vi "test_TrajectoryDL091126GenericVoxel.vi"() -> ()   [LabVIEW 2010, in "TrajectoryDL091126GenericVoxel.lvclass"]
uses:
  TrajectoryDL091126GenericVoxel.lvclass
  <vilib>/Native 3D Graph/xcontrol/3DPC_SurfacePlot.xctl
  transformation_parameters.ctl
  common/classes/SpaceVector/SpaceVector/SpaceVector.lvclass
  common/enumerations/x_y_z_enumeration.ctl
  common/enumerations/functional_global_action_enum.ctl
panel:
  in  "centerButton":bool
  in  "z offset":dbl[unit](slide)
  in  "y offset":dbl[unit](slide)
  in  "x offset":dbl[unit](slide)
  in  "number of voxels":i32=20
  in  "createPixelsButton":bool
  in  "equallyDistributeButton":bool
  out "time needed [ms]":u32
  in  "tilt angle":dbl[unit](slide)
  in  "rotation angle":dbl[unit](slide)
  in  "scale factor":dbl(slide)=1.0 scale=1.0..10.0
  out "3D Graph":refnum<class "Base Datatype.lvclass">[](xcontrol)
  in  "stopButton":bool
  # "Test Suite for TrajectoryDL091126GenericVoxel"
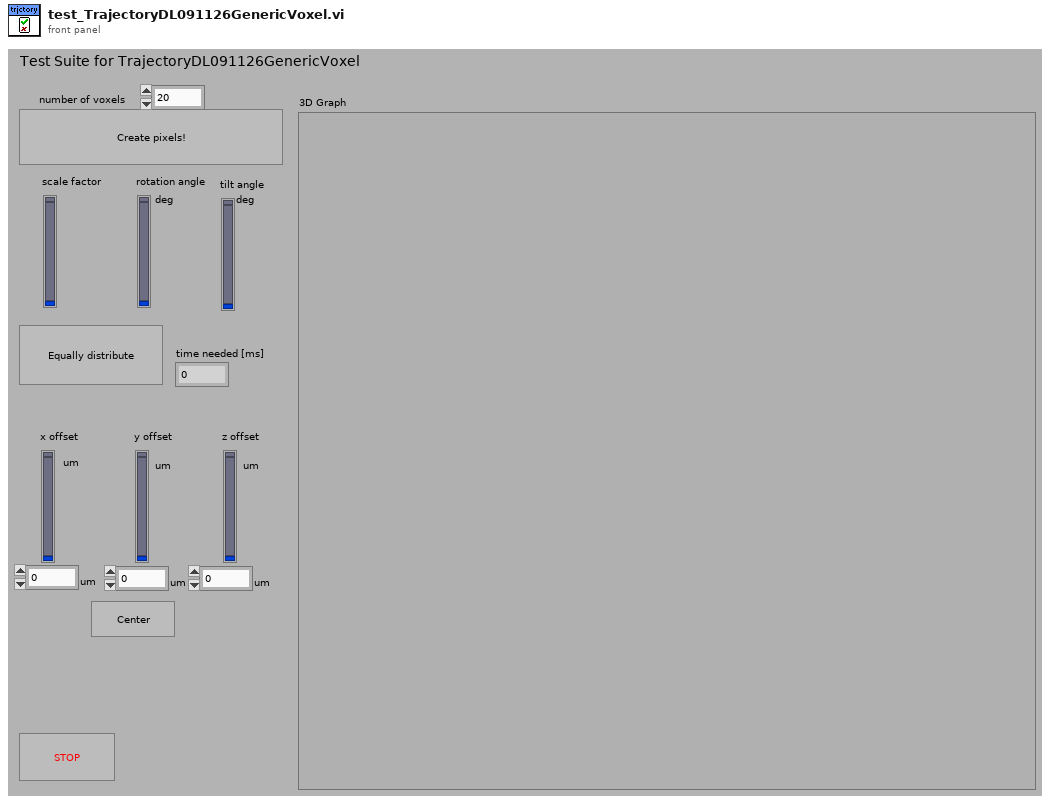
[diagram p1: front panel]
types:
  T1 = typedef "functional_global_action_enum.ctl" = enum16{"get", "set", "reset"}
  T2 = typedef "x_y_z_enumeration.ctl" = enum16{"x", "y", "z"}
  T3 = typedef "TrajectoryDL091126GenericVoxel.lvclass/transformation_parameters.ctl" = cluster{"scale factor":dbl, "rotation angle":dbl[unit], "tilting angle":dbl[unit], "offset":refnum<class "SpaceVector.lvclass">}
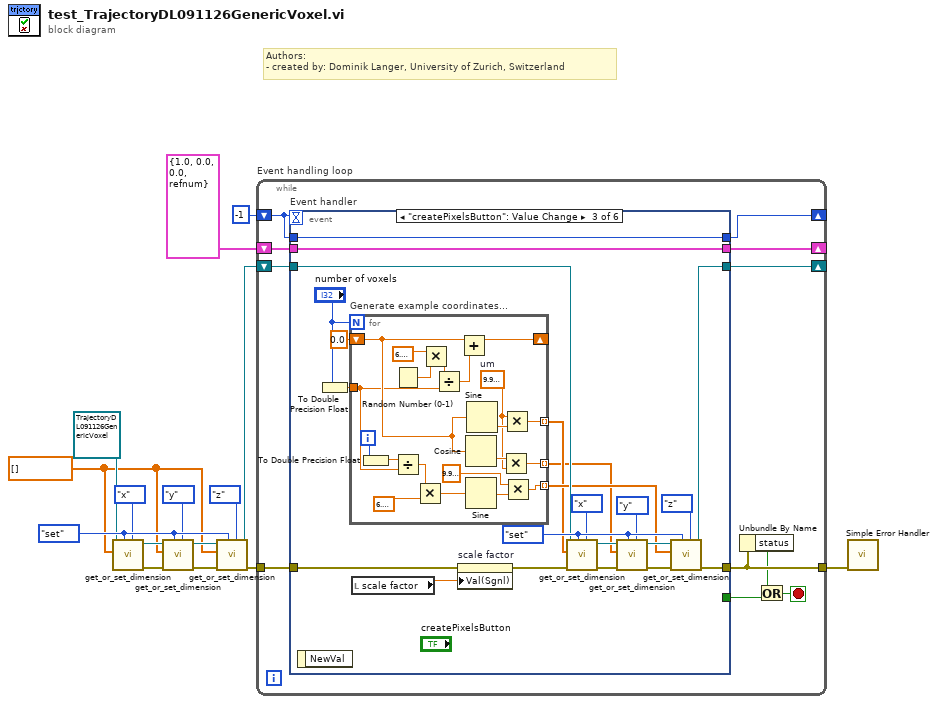
[diagram p0: block diagram]
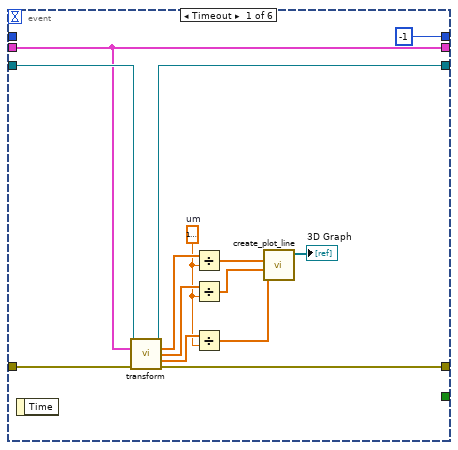
[diagram p2: hidden frame]
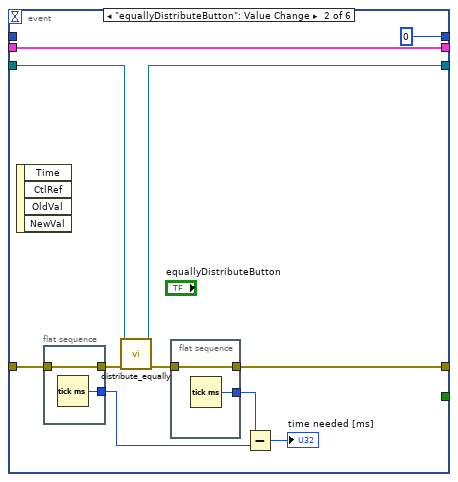
[diagram p3: hidden frame]
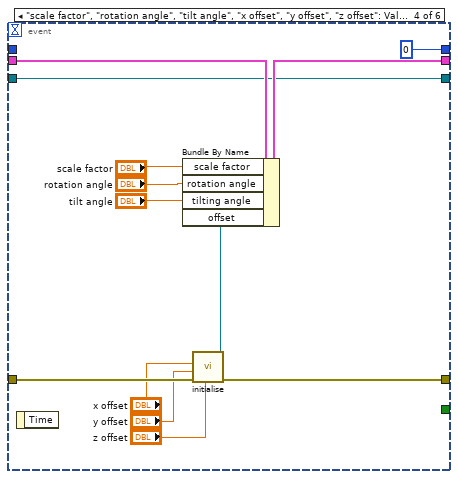
[diagram p4: hidden frame]
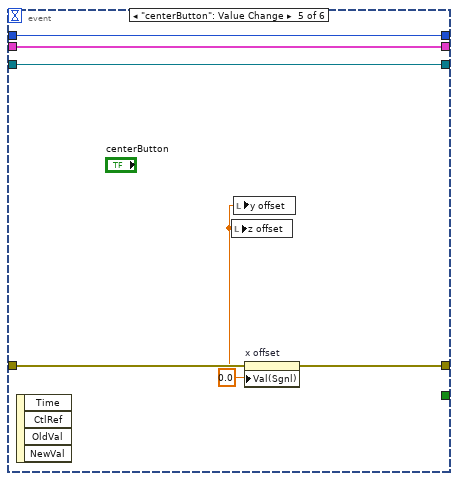
[diagram p5: hidden frame]
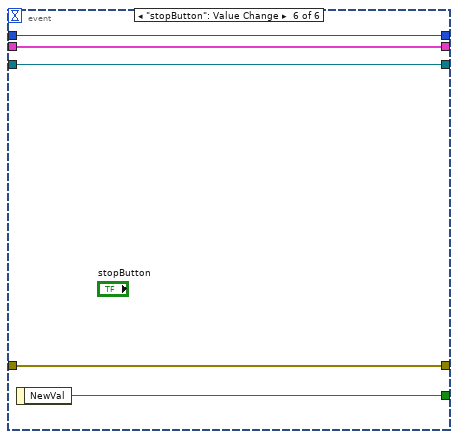
[diagram p6: hidden frame]
diagram:
  w5 = dbl[unit][] [] ("pixel values in (single dimension)")
  w13 = functional_global_action_enum."set" ("action")
  # "Authors: \n- created by: Dominik Langer, University of Zurich, Switzerland"
  n1 = call-dynamic "get_or_set_dimension.vi"("dimension"=x_y_z_enumeration."x", "action"=w13, "pixel values in (single dimension)"=w5, "GenericTrajectory in"=refnum<class "TrajectoryDL091126GenericVoxel.lvclass"> refnum) -> ("error out"=w11:errorcluster, "GenericTrajectory out"=w12:refnum<class "TrajectoryDL091126GenericVoxel.lvclass">)  [unwired: 5 in, 1 out]
  n2 = call-dynamic "get_or_set_dimension.vi"("dimension"=x_y_z_enumeration."y", "action"=w13, "error in (no error)"=w11, "pixel values in (single dimension)"=w5, "GenericTrajectory in"=w12) -> ("error out"=w9:errorcluster, "GenericTrajectory out"=w10:refnum<class "TrajectoryDL091126GenericVoxel.lvclass">)  [unwired: 4 in, 1 out]
  n3 = call-dynamic "get_or_set_dimension.vi"("dimension"=x_y_z_enumeration."z", "action"=w13, "error in (no error)"=w9, "pixel values in (single dimension)"=w5, "GenericTrajectory in"=w10) -> ("error out"=w8:errorcluster, "GenericTrajectory out"=w6:refnum<class "TrajectoryDL091126GenericVoxel.lvclass">)  [unwired: 4 in, 1 out]
  n4 = while "Event handling loop" {
    shift-right: [w25] -> _
    shift-left: -1 -> [w26]
    shift-right: [w22] -> _
    shift-left: w6 -> [w23]
    shift-right: [w20] -> _
    shift-left: T3 {"scale factor"=1.0, "rotation angle"=0.0, "tilting angle"=0.0, "offset"=refnum} ("transformation parameters") -> [w21]
    tunnel: w8 -> [w24]
    tunnel: [w17] -> w1
    stop <- w18 stop-if-true
    n5 = event "Event handler" shown="[2] \"createPixelsButton\": Value Change" {
      selector: _ -> [_ _ _ _ _ _]
      dyn-events: _ -> [_ _ _ _ _ _]
      timeout: w26 -> [_ _ _ _ _ _]
      tunnel: [-1 0 w59 0 w116 w121] -> w25
      tunnel: w26 -> [_ _ w59 _ w116 w121]
      tunnel: w24 -> [w38 w47 w58 w103 w113 w119]
      tunnel: [w37 w44 w66 w102 w112 w119] -> w17
      tunnel: [_ _ _ _ _ w120] -> w19
      tunnel: w23 -> [w36 w50 w65 w104 w115 w117]
      tunnel: [w35 w49 w64 w104 w115 w117] -> w22
      tunnel: w21 -> [w34 w51 w77 w110 w114 w118]
      tunnel: [w34 w51 w77 w109 w114 w118] -> w20
      event Timeout {
        w30 = dbl[unit] 1e-06  # um
        n6 = event-data() -> ()  [unwired: 1 in, 1 out]
        n7 = call-dynamic "transform.vi"("GenericTrajectory in"=w36, "transformation parameters"=w34, "error in (no error)"=w38) -> ("GenericTrajectory out"=w35:refnum<class "TrajectoryDL091126GenericVoxel.lvclass">, "x coordinates"=w33:dbl[unit][], "y coordinates"=w32:dbl[unit][], "z coordinates"=w31:dbl[unit][], "error out"=w37:errorcluster)  [unwired: 8 in]
        n8 = Divide(x=w33, y=w30) -> (x/y=w29:dbl[])
        n9 = Divide(x=w32, y=w30) -> (x/y=w28:dbl[])
        n10 = Divide(x=w31, y=w30) -> (x/y=w27:dbl[])
        n11 = call <vilib>:"create_plot_line.vi"("z vector"=w27, "y vector"=w28, "x vector"=w29) -> ("plots out"=→"3D Graph":refnum<class "Base Datatype.lvclass">[])  [unwired: 2 in, 6 out]
      }
      event "equallyDistributeButton": Value Change {
        n12 = event-data() -> ()  [unwired: 1 in, 4 out]
        n13 = flat-sequence {
          tunnel: w47 -> [w55]
          tunnel: [w55] -> w46
          tunnel: [w54] -> w42
          frame #0 {
            n14 = Tick Count (ms)() -> (millisecond timer value=w54:u32)
          }
        }
        n15 = call-dynamic "distribute_equally.vi"("error in (no error)"=w46, "TrajectoryDL091126GenericVoxel in"=w50) -> ("error out"=w45:errorcluster, "TrajectoryDL091126GenericVoxel out"=w49:refnum<class "TrajectoryDL091126GenericVoxel.lvclass">)  [unwired: 7 in, 1 out]
        n16 = flat-sequence {
          tunnel: w45 -> [w53]
          tunnel: [w53] -> w44
          tunnel: [w52] -> w43
          frame #0 {
            n17 = Tick Count (ms)() -> (millisecond timer value=w52:u32)
          }
        }
        n18 = Subtract(x=w43, y=w42) -> (x-y=→"time needed [ms]":u32)
      }
      event "createPixelsButton": Value Change {
        w74 = functional_global_action_enum."set" ("action")
        n19 = event-data() -> ()  [unwired: 1 in, 1 out]
        n20 = To Double Precision Float(number="number of voxels") -> (double precision float=w75:dbl)
        n21 = for "Generate example coordinates..." {
          N: "number of voxels" -> [_]
          tunnel: [w96] -> w60 mode=indexing
          tunnel: [w95] -> w61 mode=indexing
          tunnel: w75 -> [w81]
          shift-right: [w91] -> _
          shift-left: 0.0 -> [w86]
          tunnel: [w87] -> w62 mode=indexing
          i -> [w83]
          w85 = dbl[unit] 9.999999999999999e-05  # um
          n22 = To Double Precision Float(number=w83) -> (double precision float=w82:dbl)
          n23 = Random Number (0-1)() -> (number: 0 to 1=w93:dbl)
          n24 = Divide(x=w82, y=w81) -> (x/y=w79:dbl)
          n25 = Multiply(x=w79, y=6.283185307179586) -> (x*y=w78:dbl)
          n26 = Multiply(x=6.283185307179586, y=w93) -> (x*y=w92:dbl)
          n27 = Divide(x=w92, y=w81) -> (x/y=w90:dbl)
          n28 = Add(x=w86, y=w90) -> (x+y=w91:dbl)
          n29 = Cosine(x=w86) -> (cos(x)=w94:dbl)
          n30 = Sine(x=w78) -> (sin(x)=w88:dbl)
          n31 = Sine(x=w86) -> (sin(x)=w97:dbl)
          n32 = Multiply(x=w94, y=w85) -> (x*y=w96:dbl[unit])
          n33 = Multiply(x=w85, y=w97) -> (x*y=w95:dbl[unit])
          n34 = Multiply(x=dbl[unit] 9.999999999999999e-06, y=w88) -> (x*y=w87:dbl[unit])
        }
        n35 = local read "scale factor"() -> (w56:dbl)
        n36 = property on="scale factor" class="Slide (strict)"(error in=w58, "Val(Sgnl)"=w56) -> (error out=w57:errorcluster)  [unwired: 1 in, 1 out]
        n37 = call-dynamic "get_or_set_dimension.vi"("dimension"=x_y_z_enumeration."x", "action"=w74, "error in (no error)"=w57, "pixel values in (single dimension)"=w61, "GenericTrajectory in"=w65) -> ("error out"=w69:errorcluster, "GenericTrajectory out"=w70:refnum<class "TrajectoryDL091126GenericVoxel.lvclass">)  [unwired: 4 in, 1 out]
        n38 = call-dynamic "get_or_set_dimension.vi"("dimension"=x_y_z_enumeration."y", "action"=w74, "error in (no error)"=w69, "pixel values in (single dimension)"=w60, "GenericTrajectory in"=w70) -> ("error out"=w67:errorcluster, "GenericTrajectory out"=w68:refnum<class "TrajectoryDL091126GenericVoxel.lvclass">)  [unwired: 4 in, 1 out]
        n39 = call-dynamic "get_or_set_dimension.vi"("dimension"=x_y_z_enumeration."z", "action"=w74, "error in (no error)"=w67, "pixel values in (single dimension)"=w62, "GenericTrajectory in"=w68) -> ("error out"=w66:errorcluster, "GenericTrajectory out"=w64:refnum<class "TrajectoryDL091126GenericVoxel.lvclass">)  [unwired: 4 in, 1 out]
      }
      event "scale factor", "rotation angle", "tilt angle", "x offset", "y offset", "z offset": Value Change {
        n40 = event-data() -> ()  [unwired: 1 in, 1 out]
        n41 = call "initialise.vi"("z"="z offset", "error in (no error)"=w103, "y"="y offset", "x"="x offset") -> ("error out"=w102:errorcluster, "SpaceVector out"=w101:refnum<class "SpaceVector.lvclass">)  [unwired: 6 in]
        n42 = Bundle By Name(cluster=w110, "scale factor"="scale factor", "rotation angle"="rotation angle", "tilting angle"="tilt angle", "offset"=w101) -> (w109:T3)
      }
      event "centerButton": Value Change {
        w111 = dbl[unit] 0.0 ("Value (Signaling)")
        n43 = event-data() -> ()  [unwired: 1 in, 4 out]
        n44 = local write "z offset"(w111) -> ()
        n45 = local write "y offset"(w111) -> ()
        n46 = property on="x offset" class="Slide (strict)"(error in=w113, "Val(Sgnl)"=w111) -> (error out=w112:errorcluster)  [unwired: 1 in, 1 out]
      }
      event "stopButton": Value Change {
        n47 = event-data() -> ("NewVal"=w120:bool)  [unwired: 1 in]
      }
    }
    n48 = Unbundle By Name(w17) -> ("status"=w16:bool)
    n49 = Or(x=w16, y=w19) -> (x .or. y?=w18:bool)
  }
  n50 = call <vilib>:"Simple Error Handler.vi"("error in (no error)"=w1) -> ()  [unwired: 4 in, 5 out]
